vi "EyeAngleProcess.vi"(7 "method":enum16{"pupil", "CR", "pupil-CR"}(ring), 8 "valid fit":T3={"CR Valid Fit"=TRUE, "pupil Valid Fit"=TRUE}, 9 "ScaleArray":T1, 10 "AdjustFactor":T2, 11 "EYEDateArray":dbl[](array[numeric])=[0.0, 0.0]) -> (2 "ScaleIndex":i32, 3 "EyeAngle":dbl[](array[numeric]))   [LabVIEW 2011]
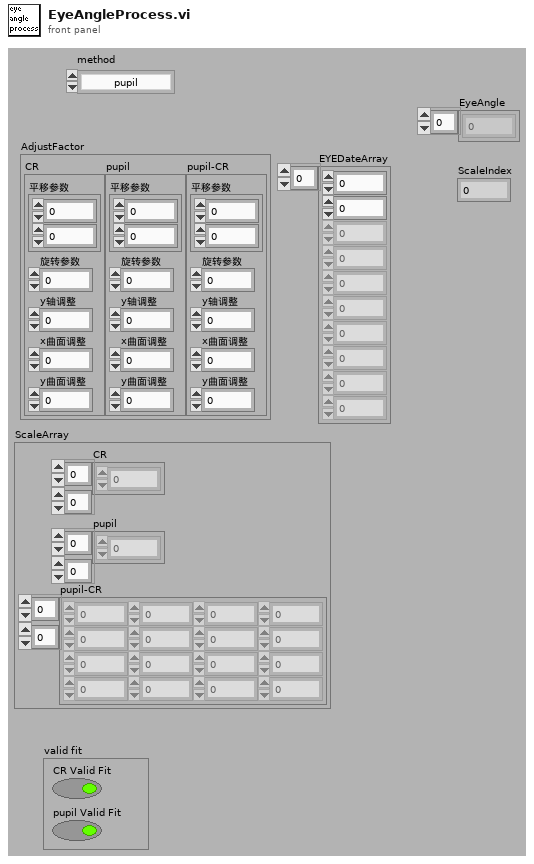
[diagram p1: front panel]
types:
  T1 = cluster{"CR":dbl[][], "pupil":dbl[][], "pupil-CR":dbl[][]}
  T2 = cluster{"CR":cluster{"平移参数":cluster{dbl, dbl}, "旋转参数":dbl, "y轴调整":dbl, "x曲面调整":dbl, "y曲面调整":dbl}, "pupil":cluster{"平移参数":cluster{dbl, dbl}, "旋转参数":dbl, "y轴调整":dbl, "x曲面调整":dbl, "y曲面调整":dbl}, "pupil-CR":cluster{"平移参数":cluster{dbl, dbl}, "旋转参数":dbl, "y轴调整":dbl, "x曲面调整":dbl, "y曲面调整":dbl}}
  T3 = cluster{"CR Valid Fit":bool, "pupil Valid Fit":bool}
  T4 = cluster{"平移参数":cluster{dbl, dbl}, "旋转参数":dbl, "y轴调整":dbl, "x曲面调整":dbl, "y曲面调整":dbl}
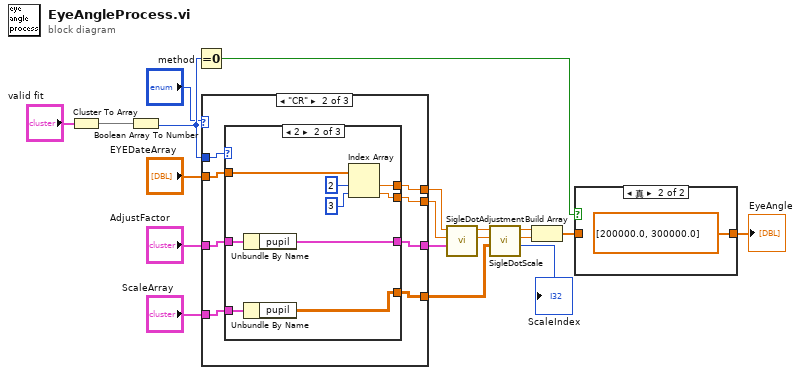
[diagram p0: block diagram]
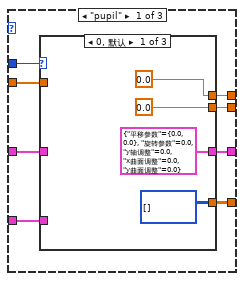
[diagram p2: hidden frame]
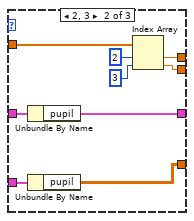
[diagram p3: hidden frame]
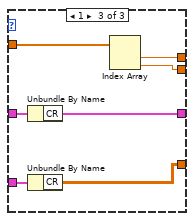
[diagram p4: hidden frame]
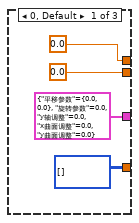
[diagram p5: hidden frame]
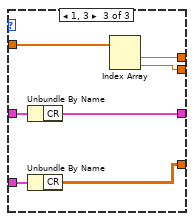
[diagram p6: hidden frame]
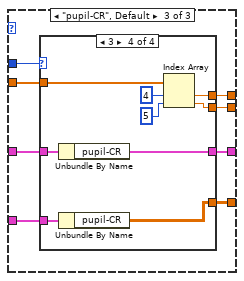
[diagram p7: hidden frame]
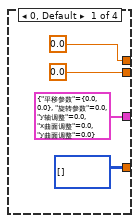
[diagram p8: hidden frame]
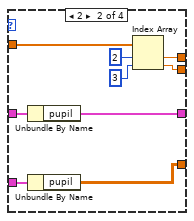
[diagram p9: hidden frame]
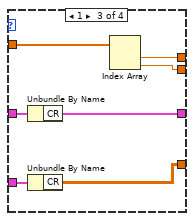
[diagram p10: hidden frame]
diagram:
  n1 = Cluster To Array(cluster="valid fit") -> (array=w18:bool[])
  n2 = Boolean Array To Number(Boolean array=w18) -> (number=w9:u32)
  n3 = Equal To 0?(x=w9) -> (x = 0?=w10:bool)
  n4 = case shown="\"CR\"" "method" {
    tunnel: "AdjustFactor" -> [w26 w50 w83]
    tunnel: "ScaleArray" -> [w25 w49 w82]
    tunnel: "EYEDateArray" -> [w27 w51 w81]
    tunnel: [w23 w55 w78] -> w5
    tunnel: [w22 w54 w77] -> w4
    tunnel: [w21 w52 w80] -> w14
    tunnel: w9 -> [w24 w48 w79]
    tunnel: [w20 w53 w76] -> w6
    frame "pupil" {
      n5 = case shown="0, 默认" w24 {
        tunnel: [T4 {"平移参数"={0.0, 0.0}, "旋转参数"=0.0, "y轴调整"=0.0, "x曲面调整"=0.0, "y曲面调整"=0.0} ("pupil-CR") w38 w46] -> w20
        tunnel: [i32[][] [] ("pupil-CR") w37 w44] -> w21
        tunnel: w26 -> [_ w40 w47]
        tunnel: w25 -> [_ w39 w45]
        tunnel: w27 -> [_ w36 w43]
        tunnel: [0.0 ("Pos. Y") w35 w42] -> w23
        tunnel: [0.0 ("Pos. Y") w34 w41] -> w22
        frame 0, Default {
        }
        frame 2, 3 {
          n6 = Unbundle By Name(w40) -> ("pupil"=w38:T4)
          n7 = Unbundle By Name(w39) -> ("pupil"=w37:dbl[][])
          n8 = Index Array(array=w36, index #1=2 ("索引"), index #2=3 ("索引")) -> (element #1=w35:dbl, element #2=w34:dbl)
        }
        frame 1 {
          n9 = Unbundle By Name(w47) -> ("CR"=w46:T4)
          n10 = Unbundle By Name(w45) -> ("CR"=w44:dbl[][])
          n11 = Index Array(array=w43) -> (element #1=w42:dbl, element #2=w41:dbl)  [unwired: 2 in]
        }
      }
    }
    frame "CR" {
      n12 = case shown="2" w48 {
        tunnel: [T4 {"平移参数"={0.0, 0.0}, "旋转参数"=0.0, "y轴调整"=0.0, "x曲面调整"=0.0, "y曲面调整"=0.0} ("pupil-CR") w66 w74] -> w53
        tunnel: [i32[][] [] ("pupil-CR") w65 w72] -> w52
        tunnel: w50 -> [_ w68 w75]
        tunnel: w49 -> [_ w67 w73]
        tunnel: w51 -> [_ w64 w71]
        tunnel: [0.0 ("Pos. Y") w63 w70] -> w55
        tunnel: [0.0 ("Pos. Y") w62 w69] -> w54
        frame 0, Default {
        }
        frame 2 {
          n13 = Unbundle By Name(w68) -> ("pupil"=w66:T4)
          n14 = Unbundle By Name(w67) -> ("pupil"=w65:dbl[][])
          n15 = Index Array(array=w64, index #1=2 ("索引"), index #2=3 ("索引")) -> (element #1=w63:dbl, element #2=w62:dbl)
        }
        frame 1, 3 {
          n16 = Unbundle By Name(w75) -> ("CR"=w74:T4)
          n17 = Unbundle By Name(w73) -> ("CR"=w72:dbl[][])
          n18 = Index Array(array=w71) -> (element #1=w70:dbl, element #2=w69:dbl)  [unwired: 2 in]
        }
      }
    }
    frame "pupil-CR", Default {
      n19 = case shown="3" w79 {
        tunnel: [T4 {"平移参数"={0.0, 0.0}, "旋转参数"=0.0, "y轴调整"=0.0, "x曲面调整"=0.0, "y曲面调整"=0.0} ("pupil-CR") w94 w102 w112] -> w76
        tunnel: [i32[][] [] ("pupil-CR") w93 w100 w111] -> w80
        tunnel: w83 -> [_ w96 w103 w110]
        tunnel: w82 -> [_ w95 w101 w109]
        tunnel: w81 -> [_ w92 w99 w106]
        tunnel: [0.0 ("Pos. Y") w91 w98 w105] -> w78
        tunnel: [0.0 ("Pos. Y") w90 w97 w104] -> w77
        frame 0, Default {
        }
        frame 2 {
          n20 = Unbundle By Name(w96) -> ("pupil"=w94:T4)
          n21 = Unbundle By Name(w95) -> ("pupil"=w93:dbl[][])
          n22 = Index Array(array=w92, index #1=2 ("索引"), index #2=3 ("索引")) -> (element #1=w91:dbl, element #2=w90:dbl)
        }
        frame 1 {
          n23 = Unbundle By Name(w103) -> ("CR"=w102:T4)
          n24 = Unbundle By Name(w101) -> ("CR"=w100:dbl[][])
          n25 = Index Array(array=w99) -> (element #1=w98:dbl, element #2=w97:dbl)  [unwired: 2 in]
        }
        frame 3 {
          n26 = Unbundle By Name(w110) -> ("pupil-CR"=w112:T4)
          n27 = Unbundle By Name(w109) -> ("pupil-CR"=w111:dbl[][])
          n28 = Index Array(array=w106, index #1=4 ("索引"), index #2=5 ("索引")) -> (element #1=w105:dbl, element #2=w104:dbl)
        }
      }
    }
  }
  n29 = call "SigleDotAdjustment.vi"("adjutFactor"=w6, "y"=w4, "x"=w5) -> ("y"=w2:dbl, "x"=w3:dbl)  [unwired: 7 out]
  n30 = call "SigleDotScale.vi"("ScaleArray"=w14, "y"=w2, "x"=w3) -> ("ScaleIndex"=→"ScaleIndex":i32, "y"=w12:dbl, "x"=w13:dbl)  [unwired: 6 out]
  n31 = Build Array(w13, w12) -> (w11:dbl[])
  n32 = case shown="真" w10 {
    tunnel: w11 -> [w113 _]
    tunnel: [w113 dbl[] [200000.0, 300000.0]] -> w8
    frame False {
    }
    frame True {
    }
  }
  "EyeAngle" <- w8
